vi "KGN Get actual Values 2.vi"(7 "scaling":dbl, 8 "Fehler (Eingang, kein Fehler)":errorcluster, 9 "Info Cluster":T1, 10 "VISA-Referenz (Eingang)":refnum<visa-resource-name>, 11 "device (Eingang)":u32) -> (0 "Fehler (Ausgang)":errorcluster, 1 "Info Cluster out":T1, 2 "VISA-Referenz (Ausgang)":refnum<visa-resource-name>, 3 "dup device (Ausgang)":u32, 4 "actual Values Cluster":T4 {"Cluster"."PumpMode-Cluster"."concentratio mode" items=["water", "reagent"]; "Cluster"."PumpMode-Cluster"."Reagent" items=["HCl", "HF", "NH3", "HG", "PPM", "ORGANIC"]}, 5 "Kommandos gesendet":string, 6 "connected":bool)   [LabVIEW 2020, in "Linearisierung v2.lvlib" / "Gasteiler.lvlib" / "HovaCAL_Interface.lvlib" / "KGN.lvlib" / "KGN GUI Get.lvlib"]
uses:
  KGN GUI Get.lvlib
  Controls/Info Cluster.ctl
  Controls/Pump Concentration Mode.ctl
  Controls/Reagent.ctl
  Controls/Controls.lvlib
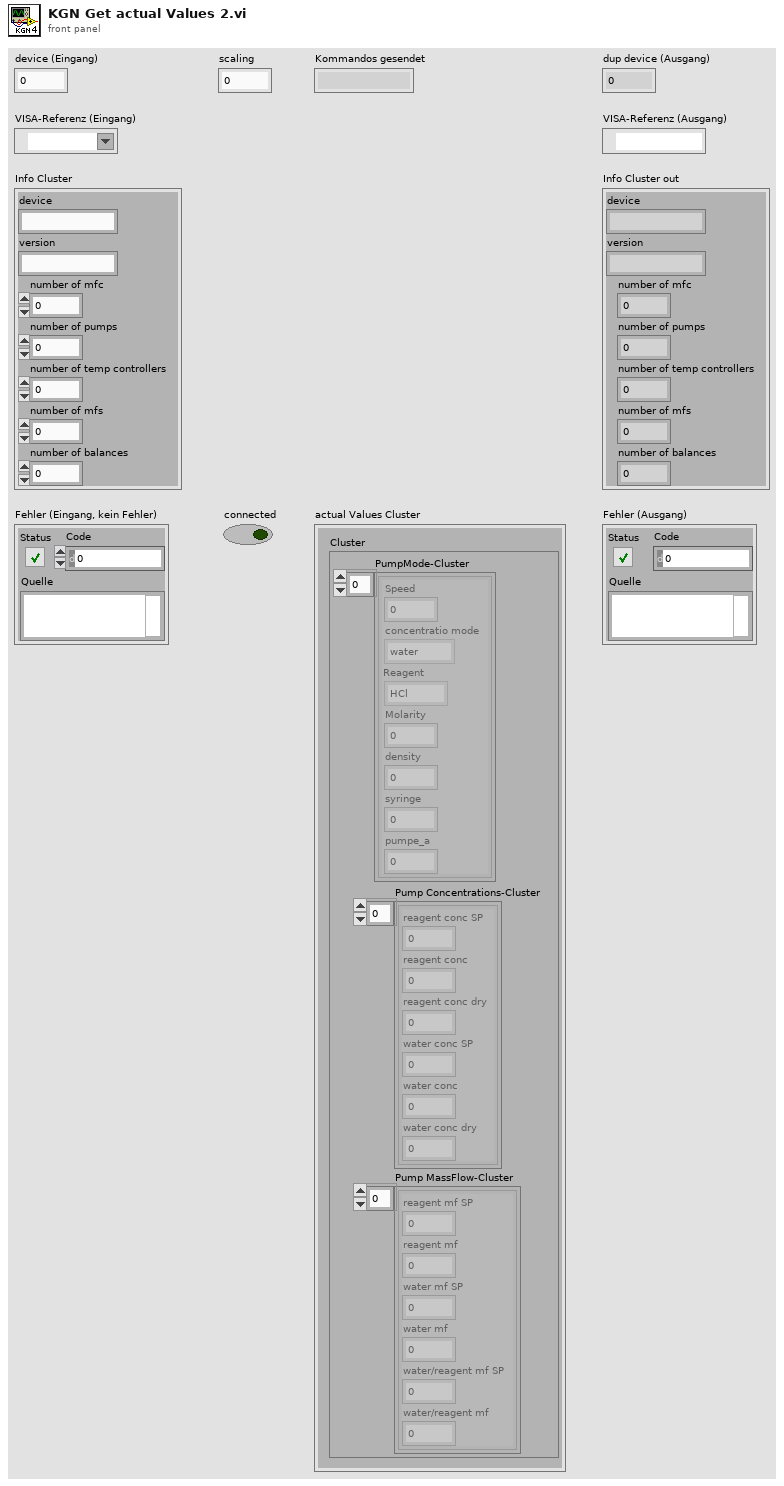
[diagram p1: front panel]
types:
  T1 = typedef "Linearisierung v2.lvlib/Gasteiler.lvlib/HovaCAL_Interface.lvlib/Controls.lvlib/Info Cluster.ctl" = cluster{"device":string, "version":string, "number of mfc":i32, "number of pumps":i32, "number of temp controllers":i32, "number of mfs":i32, "number of balances":i32}
  T2 = typedef "Linearisierung v2.lvlib/Gasteiler.lvlib/HovaCAL_Interface.lvlib/Controls.lvlib/Pump Concentration Mode.ctl" = i32
  T3 = typedef "Linearisierung v2.lvlib/Gasteiler.lvlib/HovaCAL_Interface.lvlib/Controls.lvlib/Reagent.ctl" = i32
  T4 = cluster{"Cluster":cluster{"PumpMode-Cluster":cluster{"Speed":dbl, "concentratio mode":T2, "Reagent":T3, "Molarity":dbl, "density":dbl, "syringe":dbl, "pumpe_a":dbl}[], "Pump Concentrations-Cluster":cluster{"reagent conc SP":dbl, "reagent conc":dbl, "reagent conc dry":dbl, "water conc SP":dbl, "water conc":dbl, "water conc dry":dbl}[], "Pump MassFlow-Cluster":cluster{"reagent mf SP":dbl, "reagent mf":dbl, "water mf SP":dbl, "water mf":dbl, "water/reagent mf SP":dbl, "water/reagent mf":dbl}[]}}
  T5 = cluster{"Speed":dbl, "concentratio mode":T2, "Reagent":T3, "Molarity":dbl, "density":dbl, "syringe":dbl, "pump_a":dbl}[]
  T6 = cluster{"reagent conc SP":dbl, "reagent conc":dbl, "reagent conc dry":dbl, "water conc SP":dbl, "water conc":dbl, "water conc dry":dbl}[]
  T7 = cluster{"reagent mf SP":dbl, "reagent mf":dbl, "water mf SP":dbl, "water mf":dbl, "water/reagent mf SP":dbl, "water/reagent mf":dbl}[]
  T8 = cluster{"PumpMode-Cluster":cluster{"Speed":dbl, "concentratio mode":T2, "Reagent":T3, "Molarity":dbl, "density":dbl, "syringe":dbl, "pump_a":dbl}[], "Pump Concentrations-Cluster":cluster{"reagent conc SP":dbl, "reagent conc":dbl, "reagent conc dry":dbl, "water conc SP":dbl, "water conc":dbl, "water conc dry":dbl}[], "Pump MassFlow-Cluster":cluster{"reagent mf SP":dbl, "reagent mf":dbl, "water mf SP":dbl, "water mf":dbl, "water/reagent mf SP":dbl, "water/reagent mf":dbl}[]}
  T9 = cluster{cluster{"PumpMode-Cluster":cluster{"Speed":dbl, "concentratio mode":T2, "Reagent":T3, "Molarity":dbl, "density":dbl, "syringe":dbl, "pump_a":dbl}[], "Pump Concentrations-Cluster":cluster{"reagent conc SP":dbl, "reagent conc":dbl, "reagent conc dry":dbl, "water conc SP":dbl, "water conc":dbl, "water conc dry":dbl}[], "Pump MassFlow-Cluster":cluster{"reagent mf SP":dbl, "reagent mf":dbl, "water mf SP":dbl, "water mf":dbl, "water/reagent mf SP":dbl, "water/reagent mf":dbl}[]}}
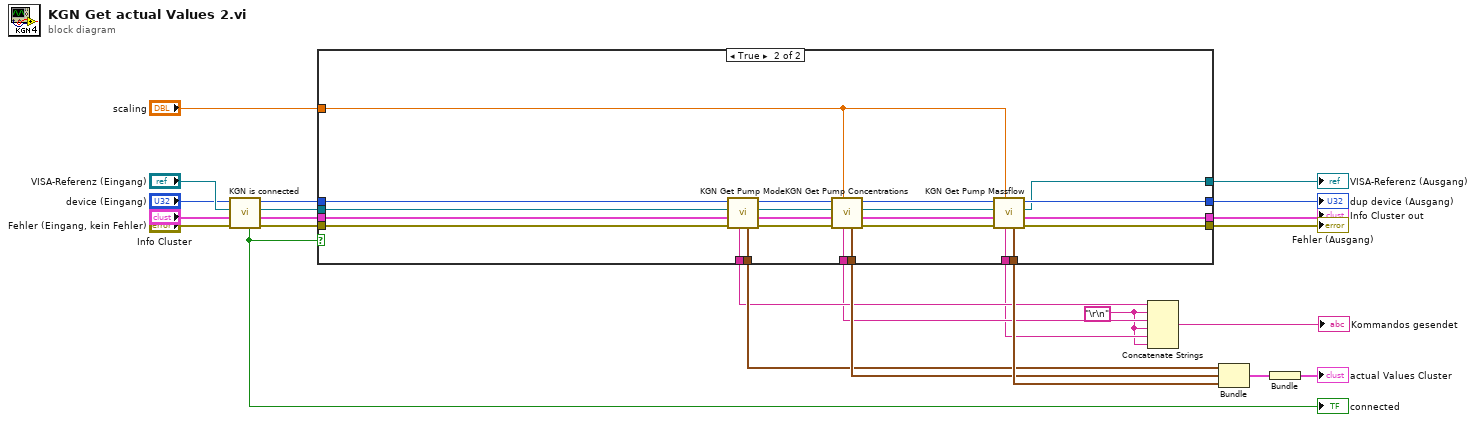
[diagram p0: block diagram]
diagram:
  w2 = "\r\n"
  n1 = call "KGN is connected.vi"("VISA-Ressourcenname"="VISA-Referenz (Eingang)", "device"="device (Eingang)") -> ("VISA-Ressourcenname out"=w21:refnum<visa-resource-name>, "dup device out"=w20:u32, "Boolesch"=w19:bool)  [unwired: 6 in, 1 out]
  "connected" <- w19
  n2 = case shown="True" w19 {
    tunnel: "Fehler (Eingang, kein Fehler)" -> [w26 w49]
    tunnel: [w26 w42] -> w10
    tunnel: w20 -> [w25 w48]
    tunnel: "Info Cluster" -> [w23 w41]
    tunnel: [w25 w43] -> w11
    tunnel: "scaling" -> [_ w32]
    tunnel: [_ w39] -> w13
    tunnel: [_ w36] -> w14
    tunnel: [_ w35] -> w17
    tunnel: w21 -> [w24 w40]
    tunnel: [w24 w31] -> w22
    tunnel: [w23 w30] -> w7
    tunnel: [_ w29] -> w5
    tunnel: [_ w28] -> w4
    tunnel: [_ w27] -> w3
    frame False {
    }
    frame True {
      n3 = call "KGN Get Pump Mode.vi"("Fehler (Eingang, kein Fehler)"=w49, "Info Cluster"=w41, "VISA-Ressourcenname"=w40, "device (Eingang)"=w48) -> ("Fehler (Ausgang)"=w46:errorcluster, "Info Cluster out"=w38:T1, "VISA-Ressourcenname out"=w37:refnum<visa-resource-name>, "dup device (Ausgang)"=w47:u32, "PumpMode-Cluster"=w39:T5, "Kommandos gesendet"=w29:string)  [unwired: 2 in]
      n4 = call "KGN Get Pump Concentrations.vi"("scaling"=w32, "Fehler (Eingang, kein Fehler)"=w46, "Info Cluster"=w38, "VISA-Ressourcenname"=w37, "device (Eingang)"=w47) -> ("Fehler (Ausgang)"=w44:errorcluster, "Info Cluster out"=w34:T1, "VISA-Ressourcenname out"=w33:refnum<visa-resource-name>, "dup device (Ausgang)"=w45:u32, "Pump Concentrations-Cluster"=w36:T6, "Kommandos gesendet"=w28:string)  [unwired: 1 in]
      n5 = call "KGN Get Pump Massflow.vi"("scaling"=w32, "Fehler (Eingang, kein Fehler)"=w44, "Info Cluster"=w34, "VISA-Referenz (Eingang)"=w33, "device (Eingang)"=w45) -> ("Fehler (Ausgang)"=w42:errorcluster, "Info Cluster out"=w30:T1, "VISA-Referenz (Ausgang)"=w31:refnum<visa-resource-name>, "dup device (Ausgang)"=w43:u32, "Pump MassFlow-Cluster"=w35:T7, "Kommandos gesendet"=w27:string)  [unwired: 1 in]
    }
  }
  "VISA-Referenz (Ausgang)" <- w22
  "dup device (Ausgang)" <- w11
  "Fehler (Ausgang)" <- w10
  "Info Cluster out" <- w7
  n6 = Concatenate Strings(w5, w2, w4, w2, w3, w2) -> (→"Kommandos gesendet":string)
  n7 = Bundle("PumpMode-Cluster"=w13, "Pump Concentrations-Cluster"=w14, "Pump MassFlow-Cluster"=w17) -> (w8:T8)  [unwired: 1 in]
  n8 = Bundle(w8) -> (→"actual Values Cluster":T9)  [unwired: 1 in]
